vi "create.vi"(8 "error in":errorcluster, 11 "mcap.channel_locator in":refnum<class "mcap.channel_locator.lvclass">) -> (0 "error out":errorcluster, 3 "mcap.channel_locator out":refnum<class "mcap.channel_locator.lvclass">)   [LabVIEW 2018, in "mcap.channel_locator.lvclass"]
uses:
  mcap.channel_locator.lvclass
  mcap.channel_locator.lvclass/mcap.channel_locator.ctl
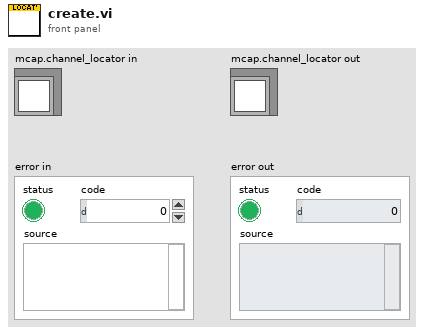
[diagram p1: front panel]
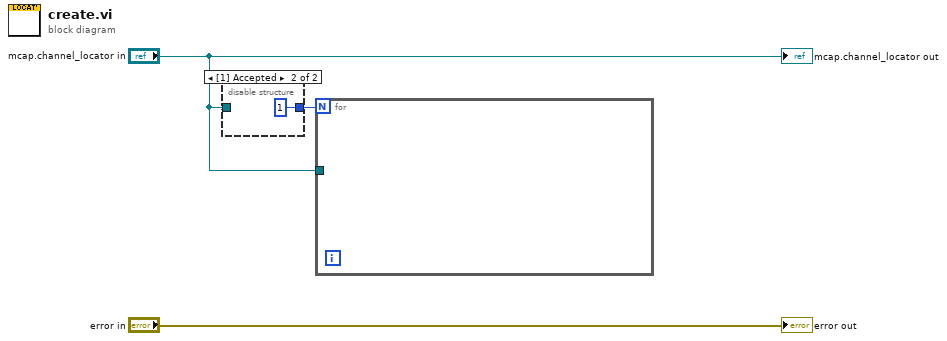
[diagram p0: block diagram]
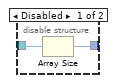
[diagram p2: hidden frame]
diagram:
  n1 = disable-structure shown="[1] Accepted" {
    disable-tunnel: "mcap.channel_locator in" -> [w5 _]
    disable-tunnel: [w4 1] -> w1
    frame Disabled {
      n2 = Array Size(array=w5) -> (size(s)=w4:i32)
    }
    frame Enabled {
    }
  }
  n3 = for {
    N: w1 -> [_]
    tunnel: "mcap.channel_locator in" -> [_]
  }
  "mcap.channel_locator out" <- "mcap.channel_locator in"
  "error out" <- "error in"
